vi "CB Holonomic Drivebase Model.vi"(11 "dt":dbl=-1.0) -> (3 "Discrete SSM":T1)   [LabVIEW 2020]
uses:
  CB State Space.ctl
  <vilib>/Analysis/Matrix/Datatypes/RealMatrix.ctl
  <vilib>/Analysis/Matrix/NI_Matrix.lvlib
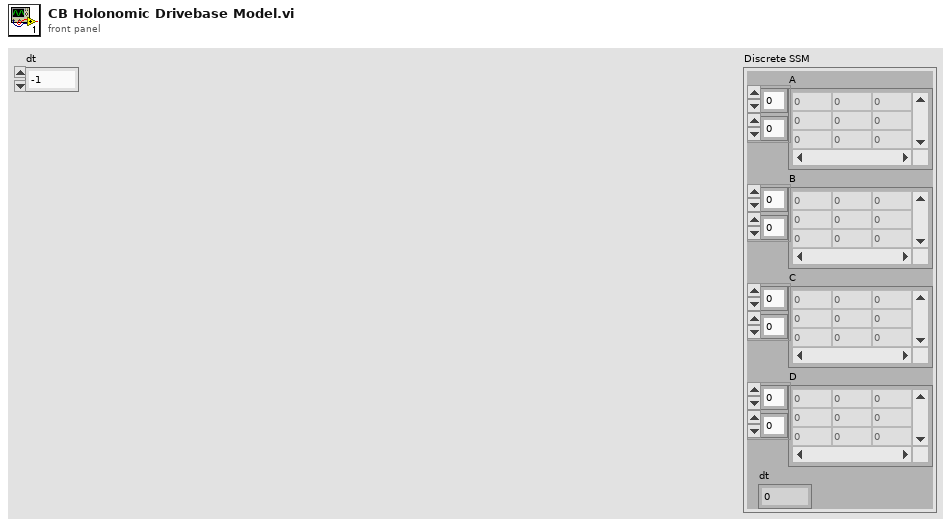
[diagram p1: front panel]
types:
  T1 = typedef "CB State Space.ctl" = cluster{"A":T2, "B":T2, "C":T2, "D":T2, "dt":dbl}
  T2 = typedef "NI_Matrix.lvlib/RealMatrix.ctl" = dbl[][]
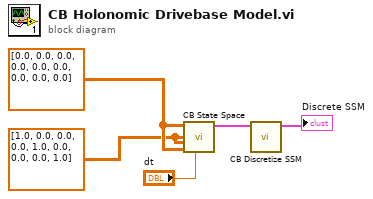
[diagram p0: block diagram]
diagram:
  w4 = T2 [[1.0, 0.0, 0.0], [0.0, 1.0, 0.0], [0.0, 0.0, 1.0]] ("resized matrix")
  w5 = T2 [[0.0, 0.0, 0.0], [0.0, 0.0, 0.0], [0.0, 0.0, 0.0]] ("resized matrix")
  n1 = call "CB State Space.vi"("dt"="dt", "D"=w5, "C"=w4, "B"=w4, "A"=w5) -> ("State Space Model"=w2:T1)  [unwired: 5 in, 1 out]
  n2 = call "CB Discretize SSM.vi"("Cont SSM"=w2) -> ("State Space Model"=→"Discrete SSM":T1)  [unwired: 10 in]
